vi "ManualLift.vi"(9 "Numeric 2":dbl, 11 "Feeder Power":dbl) -> (1 "Numeric 3":dbl, 3 "Feeder Power":dbl)   [LabVIEW 2017]
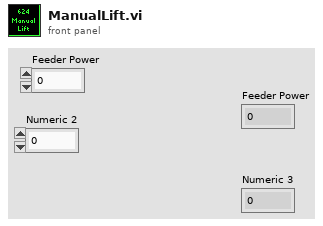
[diagram p1: front panel]
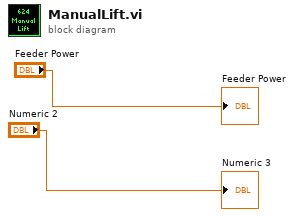
[diagram p0: block diagram]
diagram:
  "Feeder Power" <- "Feeder Power"
  "Numeric 3" <- "Numeric 2"
